vi "Instrument Type ID.vi"() -> (1 "instrument type id":string="Keysight34401A_DMM")   [LabVIEW 2020, in "Keysight 34401A DMM Instrument.lvlib"]
uses:
  Keysight 34401A DMM Instrument.lvlib
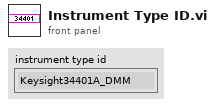
[diagram p1: front panel]
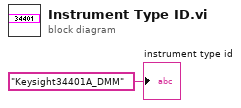
[diagram p0: block diagram]
diagram:
  "instrument type id" <- "Keysight34401A_DMM" ("instrument_type_id")
